vi "WriteSQLite.vi"(8 "error in (no error)":errorcluster, 9 "Force RMS":dbl, 10 "Torque RMS":dbl, 11 "db file":path) -> (0 "error out":errorcluster)   [LabVIEW 2020]
doc: "This VI writes to a SQLite Database the following value - Serial Number - Torque - Force"
uses:
  <vilib>/drjdpowell/SQLite Library/SQL Connection/Open (path).vi
  <vilib>/drjdpowell/SQLite Library/SQL Connection/Open (string).vi
  <vilib>/AdvancedString/Path To Command Line String.vi
  <vilib>/drjdpowell/SQLite Library/SQL Connection/Execute SQL (No results).vi
  <vilib>/drjdpowell/SQLite Library/SQL Connection/Connection.lvclass
  <vilib>/drjdpowell/SQLite Library/SQLite.lvlib
panel:
  out "resulting string":string
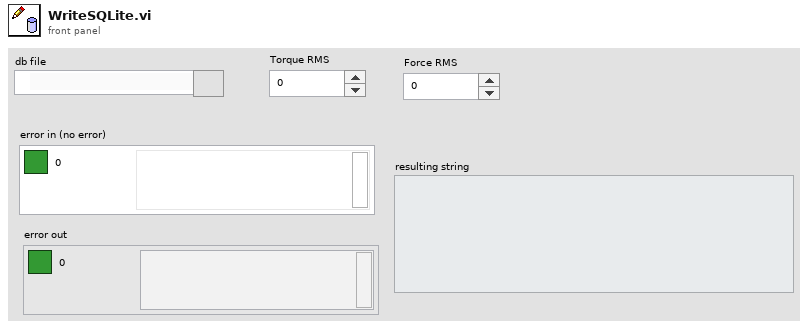
[diagram p1: front panel]
types:
  T1 = cluster{"Start Measure":bool, "Serial Number":string, "Delete Data":bool}
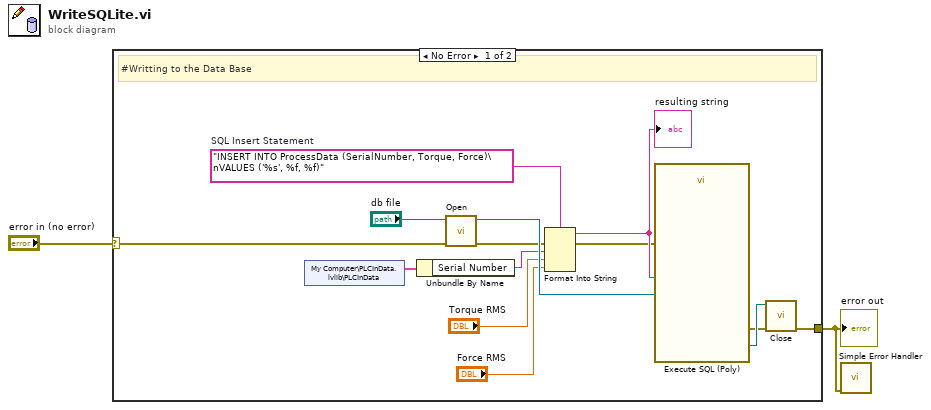
[diagram p0: block diagram]
diagram:
  n1 = case shown="No Error" "error in (no error)" {
    selector: "error in (no error)" -> [w16 w17]
    tunnel: [w5 w17] -> w1
    frame No Error {
      w11 = "INSERT INTO ProcessData (SerialNumber, Torque, Force)\nVALUES ('%s', %f, %f)"  # SQL Insert Statement
      # "#Writting to the Data Base"
      n2 = shared-variable "My Computer\\PLCInData.lvlib\\PLCInData"() -> (w4:T1)  [unwired: 1 in, 1 out]
      n3 = Unbundle By Name(w4) -> ("Serial Number"=w3:string)
      n4 = call-poly <vilib>:"Open.vi"("error in (no error)"=w16, "db file"="db file") -> ("error out"=w9:errorcluster, "SQLite Connection"=w14:refnum<class "Connection.lvclass">)  [unwired: 8 in]
      n5 = Format Into String "Format Into String"(format string=w11, error in=w9, w3, "Torque RMS", "Force RMS") -> (resulting string=w10:string, error out=w8:errorcluster)  [unwired: 1 in]
      "resulting string" <- w10
      n6 = call-poly <vilib>:"Execute SQL (Poly).vi"("error in (no error)"=w8, "SQL"=w10, "SQLite Connection in"=w14) -> ("error out"=w6:errorcluster, "SQLite Connection"=w7:refnum<class "Connection.lvclass">)  [unwired: 7 in]
      n7 = call-dynamic "Close.vi"("error in (no error)"=w6, "SQLite Connection in"=w7) -> ("error out"=w5:errorcluster)  [unwired: 9 in]
    }
    frame Error {
    }
  }
  "error out" <- w1
  n8 = call <vilib>:"Simple Error Handler.vi"("error in (no error)"=w1) -> ()  [unwired: 4 in, 5 out]
